vi "Set PDOMapping.vi"(8 "error in":errorcluster, 10 "PDOMapping":refnum<class "Value.lvclass">, 11 "DOMAIN in":refnum<class "DOMAIN.lvclass">) -> (0 "error out":errorcluster, 3 "DOMAIN out":refnum<class "DOMAIN.lvclass">)   [LabVIEW 2024, in "Electronic Datasheet.lvlib" / "DOMAIN.lvclass"]
uses:
  DOMAIN.lvclass
  Value/Value.lvclass
  Electronic Datasheet.lvlib
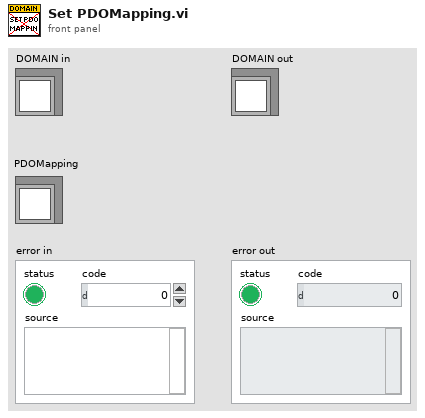
[diagram p1: front panel]
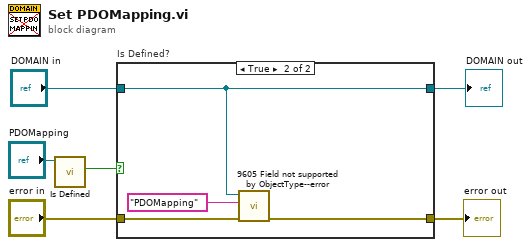
[diagram p0: block diagram]
diagram:
  n1 = call "Is Defined.vi"("Value in"="PDOMapping") -> ("Is Defined?"=w2:bool)  [unwired: 9 in, 1 out]
  n2 = case "Is Defined?" shown="True" w2 {
    tunnel: "error in" -> [w8 w12]
    tunnel: [w8 w11] -> w5
    tunnel: "DOMAIN in" -> [w7 w9]
    tunnel: [w7 w9] -> w1
    frame False {
    }
    frame True {
      n3 = call "9605 Field not supported by ObjectType--error.vi"("error in"=w12, "Field Name"="PDOMapping" ("Field name"), "Object Type Base"=w9) -> ("error out"=w11:errorcluster)  [unwired: 8 in]
    }
  }
  "DOMAIN out" <- w1
  "error out" <- w5
